vi "Split Control FPGA cluster.vi"(10 "New DAQ FPGA Configuration":T6={"Target"="RIO0", "input card type"=enum."AC Card", "Ref"=refnum, "Clock Freq (MHz) "=200.0, "Samples Wait after Trigger"=5080, "AOD fill"=4900, "StartupDelay"=0, "Slip Cycle (clock cycles)"=600000, "Add Cycle"=TRUE}, 11 "New Control FPGA Configuration":T7={"Contrl Sys Available Ind"=FALSE, "Control system.FPGA Type"=enum."Virtex 5", "Control system.Network adapter name"="", "Control system.MAC address"="", "Control system.Ethernet Port"=3, "Ethernet opened"=FALSE, "Ctrl FPGA Clock (MHz)"=240.0, "AOD 1 Amplitude"=0, "AOD 2 Amplitude"=0, "AOD 3 Amplitude"=0, "AOD 4 Amplitude"=0, "AOD 5 Amplitude"=0, "AOD 6 Amplitude"=0, "Data Time Interval (ns)"=0.0, "T0 (ns)"=0.0, "Ta (ns)"=0.0} {"Control system.Ethernet Port" min=0 max=2048 step=1; "Ctrl FPGA Clock (MHz)" min=80.0 max=500.0 step=1.0; "Data Time Interval (ns)" min=0.0 max=2048.0 step=1.0; "Ta (ns)" min=0.0 max=2048.0 step=1.0; "T0 (ns)" min=0.0 max=2048.0 step=1.0; "AOD 6 Amplitude" min=0 max=2048 step=1; "AOD 5 Amplitude" min=0 max=2048 step=1; "AOD 4 Amplitude" min=0 max=2048 step=1; "AOD 3 Amplitude" min=0 max=2048 step=1; "AOD 2 Amplitude" min=0 max=2048 step=1; "AOD 1 Amplitude" min=0 max=2048 step=1}) -> (0 "DAQ FPGA System Config":T5={"Clock Freq (MHz) "=200.0, "Samples Wait after Trigger"=5080, "AOD fill"=4900, "StartupDelay"=0, "Slip Cycle (clock cycles)"=600000, "Add Cycle"=TRUE}, 1 "Control FPGA System Config":T8={"AOD 1 Amplitude"=0, "AOD 2 Amplitude"=0, "AOD 3 Amplitude"=0, "AOD 4 Amplitude"=0, "AOD 5 Amplitude"=0, "AOD 6 Amplitude"=0, "T0 (ns)"=0.0, "Ta (ns)"=0.0, "Data Time Interval (ns)"=0.0, "Ctrl FPGA Clock (MHz)"=240.0} {"Ctrl FPGA Clock (MHz)" min=80.0 max=500.0 step=1.0; "Data Time Interval (ns)" min=0.0 max=2048.0 step=1.0; "Ta (ns)" min=0.0 max=2048.0 step=1.0; "T0 (ns)" min=0.0 max=2048.0 step=1.0; "AOD 6 Amplitude" min=0 max=2048 step=1; "AOD 5 Amplitude" min=0 max=2048 step=1; "AOD 4 Amplitude" min=0 max=2048 step=1; "AOD 3 Amplitude" min=0 max=2048 step=1; "AOD 2 Amplitude" min=0 max=2048 step=1; "AOD 1 Amplitude" min=0 max=2048 step=1}, 2 "DAQ FPGA HW Config":T1={"FGPA Ref"=refnum, "Target"="RIO0", "input card type"=enum."AC Card"}, 3 "Control FPGA HW Config":T9, 5 "Contrl Sys Available Ind":bool)   [LabVIEW 2017]
uses:
  Typedefs/Control Sys HW config cluster.ctl
  Typedefs/CTRL system config.ctl
  Typedefs/CTRL system config cluster.ctl
  Typedefs/DAQ FPGA config cluster.ctl
  <vilib>/userdefined/High Color/nirio_resource_hc.ctl
  Typedefs/FPGA input type AC-DC.ctl
  RIG-SPECIFIC FILES/FPGA Refs/FPGA Ref.ctl
  Typedefs/DAQ FPGA system config.ctl
  Typedefs/DAQ FPGA HW config cluster.ctl
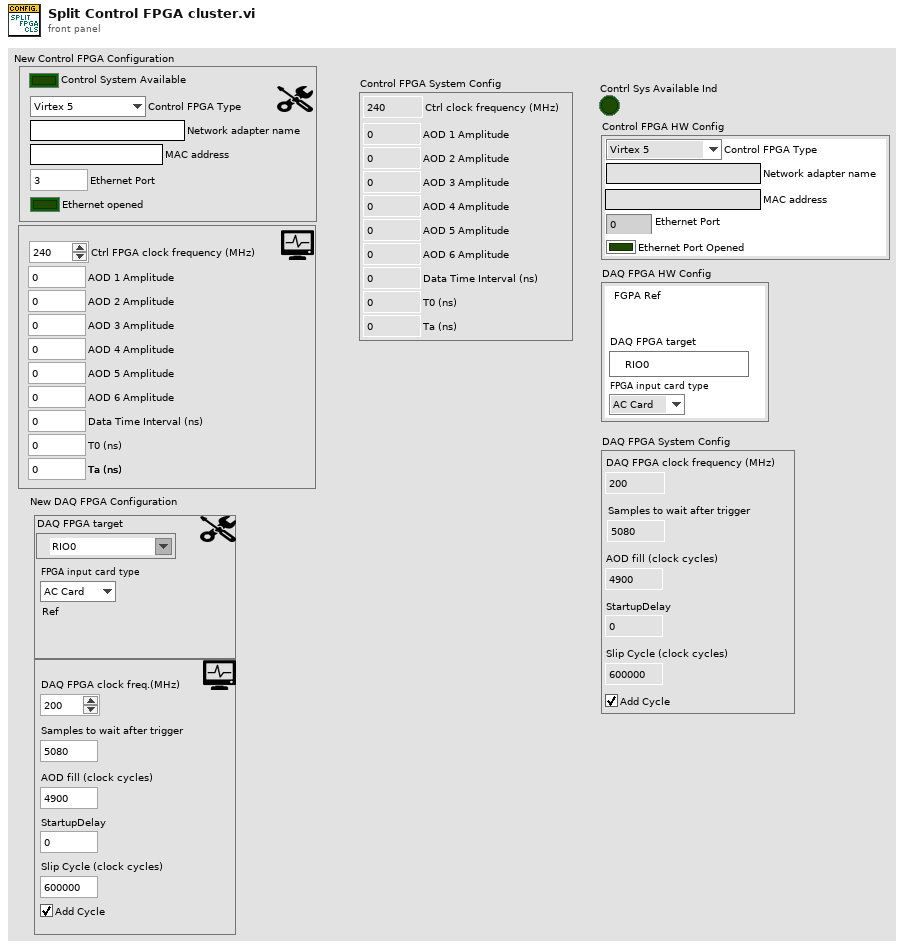
[diagram p1: front panel]
types:
  T1 = typedef "DAQ FPGA HW config cluster.ctl" = cluster{"FGPA Ref":T2, "Target":T3, "input card type":T4}
  T2 = typedef "FPGA Ref.ctl" = refnum<k20>
  T3 = typedef "nirio_resource_hc.ctl" = tag
  T4 = typedef "FPGA input type AC-DC.ctl" = enum16{"AC Card", "DC Card"}
  T5 = typedef "DAQ FPGA system config.ctl" = cluster{"Clock Freq (MHz) ":dbl, "Samples Wait after Trigger":u16, "AOD fill":u16, "StartupDelay":i32, "Slip Cycle (clock cycles)":u32, "Add Cycle":bool}
  T6 = typedef "DAQ FPGA config cluster.ctl" = cluster{"Target":T3, "input card type":T4, "Ref":T2, "Clock Freq (MHz) ":dbl, "Samples Wait after Trigger":u16, "AOD fill":u16, "StartupDelay":i32, "Slip Cycle (clock cycles)":u32, "Add Cycle":bool}
  T7 = typedef "CTRL system config cluster.ctl" = cluster{"Contrl Sys Available Ind":bool, "Control system.FPGA Type":enum16{"Virtex 5", "Virtex 7"}, "Control system.Network adapter name":string, "Control system.MAC address":string, "Control system.Ethernet Port":i16, "Ethernet opened":bool, "Ctrl FPGA Clock (MHz)":dbl, "AOD 1 Amplitude":i16, "AOD 2 Amplitude":i16, "AOD 3 Amplitude":i16, "AOD 4 Amplitude":i16, "AOD 5 Amplitude":i16, "AOD 6 Amplitude":i16, "Data Time Interval (ns)":dbl, "T0 (ns)":dbl, "Ta (ns)":dbl}
  T8 = typedef "CTRL system config.ctl" = cluster{"AOD 1 Amplitude":i16, "AOD 2 Amplitude":i16, "AOD 3 Amplitude":i16, "AOD 4 Amplitude":i16, "AOD 5 Amplitude":i16, "AOD 6 Amplitude":i16, "T0 (ns)":dbl, "Ta (ns)":dbl, "Data Time Interval (ns)":dbl, "Ctrl FPGA Clock (MHz)":dbl}
  T9 = typedef "Control Sys HW config cluster.ctl" = cluster{"Control system.FPGA Type":enum16{"Virtex 5", "Virtex 7"}, "Control system.Network adapter name":string, "Control system.MAC address":string, "Control system.Ethernet Port":u32, "Control system.Ethernet Port Opened":bool}
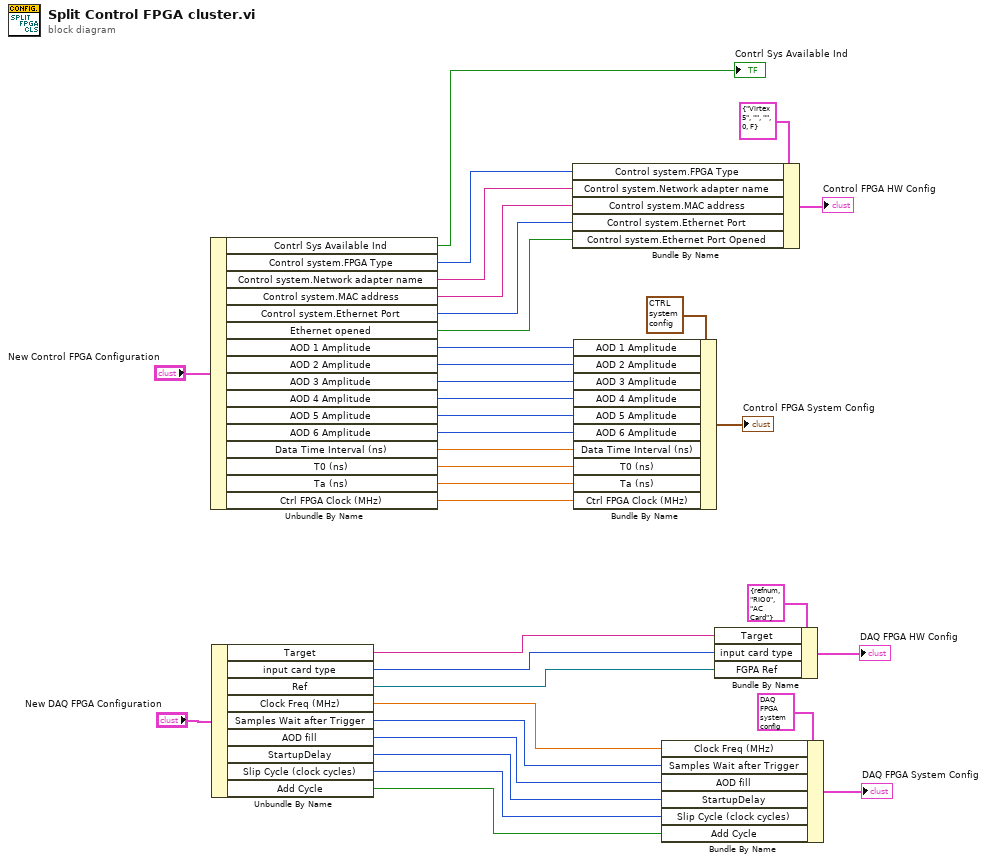
[diagram p0: block diagram]
diagram:
  n1 = Unbundle By Name("New Control FPGA Configuration") -> ("Contrl Sys Available Ind"=→"Contrl Sys Available Ind":bool, "Control system.FPGA Type"=w24:enum16{"Virtex 5", "Virtex 7"}, "Control system.Network adapter name"=w23:string, "Control system.MAC address"=w22:string, "Control system.Ethernet Port"=w5:i16, "Ethernet opened"=w1:bool, "AOD 1 Amplitude"=w35:i16, "AOD 2 Amplitude"=w34:i16, "AOD 3 Amplitude"=w33:i16, "AOD 4 Amplitude"=w32:i16, "AOD 5 Amplitude"=w31:i16, "AOD 6 Amplitude"=w30:i16, "Data Time Interval (ns)"=w29:dbl, "T0 (ns)"=w28:dbl, "Ta (ns)"=w27:dbl, "Ctrl FPGA Clock (MHz)"=w26:dbl)
  n2 = Unbundle By Name("New DAQ FPGA Configuration") -> ("Target"=w15:T3, "input card type"=w14:T4, "Ref"=w3:T2, "Clock Freq (MHz)"=w12:dbl, "Samples Wait after Trigger"=w11:u16, "AOD fill"=w10:u16, "StartupDelay"=w9:i32, "Slip Cycle (clock cycles)"=w8:u32, "Add Cycle"=w7:bool)
  n3 = Bundle By Name(cluster=T9 {"Control system.FPGA Type"=enum."Virtex 5", "Control system.Network adapter name"="", "Control system.MAC address"="", "Control system.Ethernet Port"=0, "Control system.Ethernet Port Opened"=FALSE} ("Control Sys. HW config"), "Control system.FPGA Type"=w24, "Control system.Network adapter name"=w23, "Control system.MAC address"=w22, "Control system.Ethernet Port"=w5, "Control system.Ethernet Port Opened"=w1) -> (→"Control FPGA HW Config":T9)
  n4 = Bundle By Name(cluster=T8 {"AOD 1 Amplitude"=0, "AOD 2 Amplitude"=0, "AOD 3 Amplitude"=0, "AOD 4 Amplitude"=0, "AOD 5 Amplitude"=0, "AOD 6 Amplitude"=0, "T0 (ns)"=0.0, "Ta (ns)"=0.0, "Data Time Interval (ns)"=0.0, "Ctrl FPGA Clock (MHz)"=240.0} ("Controller System Config"), "AOD 1 Amplitude"=w35, "AOD 2 Amplitude"=w34, "AOD 3 Amplitude"=w33, "AOD 4 Amplitude"=w32, "AOD 5 Amplitude"=w31, "AOD 6 Amplitude"=w30, "Data Time Interval (ns)"=w29, "T0 (ns)"=w28, "Ta (ns)"=w27, "Ctrl FPGA Clock (MHz)"=w26) -> (→"Control FPGA System Config":T8)
  n5 = Bundle By Name(cluster=T5 {"Clock Freq (MHz) "=200.0, "Samples Wait after Trigger"=5080, "AOD fill"=4900, "StartupDelay"=0, "Slip Cycle (clock cycles)"=600000, "Add Cycle"=TRUE} ("DAQ FPGA System"), "Clock Freq (MHz)"=w12, "Samples Wait after Trigger"=w11, "AOD fill"=w10, "StartupDelay"=w9, "Slip Cycle (clock cycles)"=w8, "Add Cycle"=w7) -> (→"DAQ FPGA System Config":T5)
  n6 = Bundle By Name(cluster=T1 {"FGPA Ref"=refnum, "Target"="RIO0", "input card type"=enum."AC Card"} ("DAQ FPGA HW Config"), "Target"=w15, "input card type"=w14, "FGPA Ref"=w3) -> (→"DAQ FPGA HW Config":T1)
